vi "Mean.vi"(11 "file path (dialog if empty)":path) -> (3 "Array":dbl[](array[numeric]))   [LabVIEW 2011]
uses:
  <vilib>/Utility/file.llb/Read From Spreadsheet File (DBL).vi
  <vilib>/Analysis/NI_AALBase.lvlib
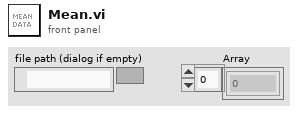
[diagram p1: front panel]
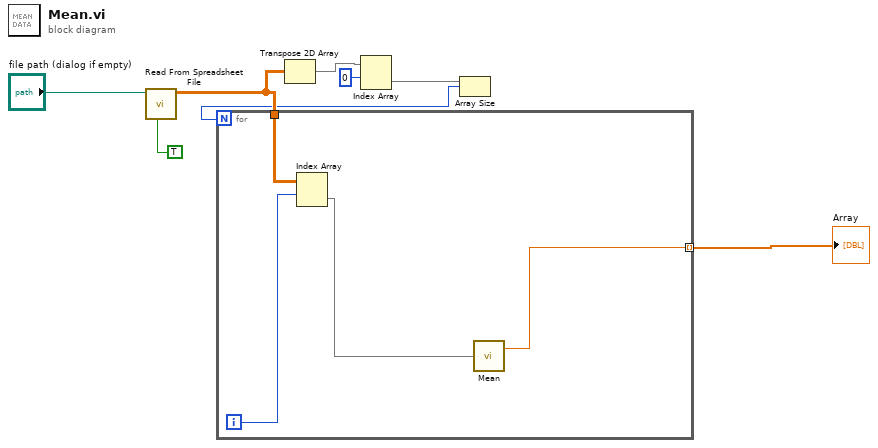
[diagram p0: block diagram]
diagram:
  n1 = call-poly <vilib>:"Read From Spreadsheet File.vi"("transpose (no:F)"=TRUE, "file path (dialog if empty)"="file path (dialog if empty)") -> ("all rows"=w6:dbl[][])  [unwired: 5 in, 4 out]
  n2 = Transpose 2D Array(2D array=w6) -> (transposed array=w7:dbl[][])
  n3 = Index Array(array=w7, index (row)=0) -> (element=w3:dbl[])  [unwired: 1 in]
  n4 = Array Size(array=w3) -> (size(s)=w4:i32)
  n5 = for {
    N: w4 -> [_]
    tunnel: w6 -> [w12]
    tunnel: [w10] -> w5 mode=indexing
    i -> [w11]
    n6 = Index Array(array=w12, index (row)=w11) -> (element=w9:dbl[])  [unwired: 1 in]
    n7 = call <vilib>:"Mean.vi"("X"=w9) -> ("mean"=w10:dbl)  [unwired: 1 out]
  }
  "Array" <- w5
